vi "Z to circle.vi"(8 "Error In":errorcluster, 10 "Plot points":i32=90, 11 "Z":cdb[](array[numeric])) -> (0 "Error Out":errorcluster, 1 "y0":dbl, 2 "x0":dbl, 3 "plot":cluster{"Array":dbl[], "Array":dbl[]}, 4 "r":dbl format="%.2f", 5 "theta":dbl)   [LabVIEW 2016]
uses:
  <vilib>/gmath/NI_Gmath.lvlib
panel:
  out "Circle fit":cluster{"Array":dbl[], "Array":dbl[]}[](graph)
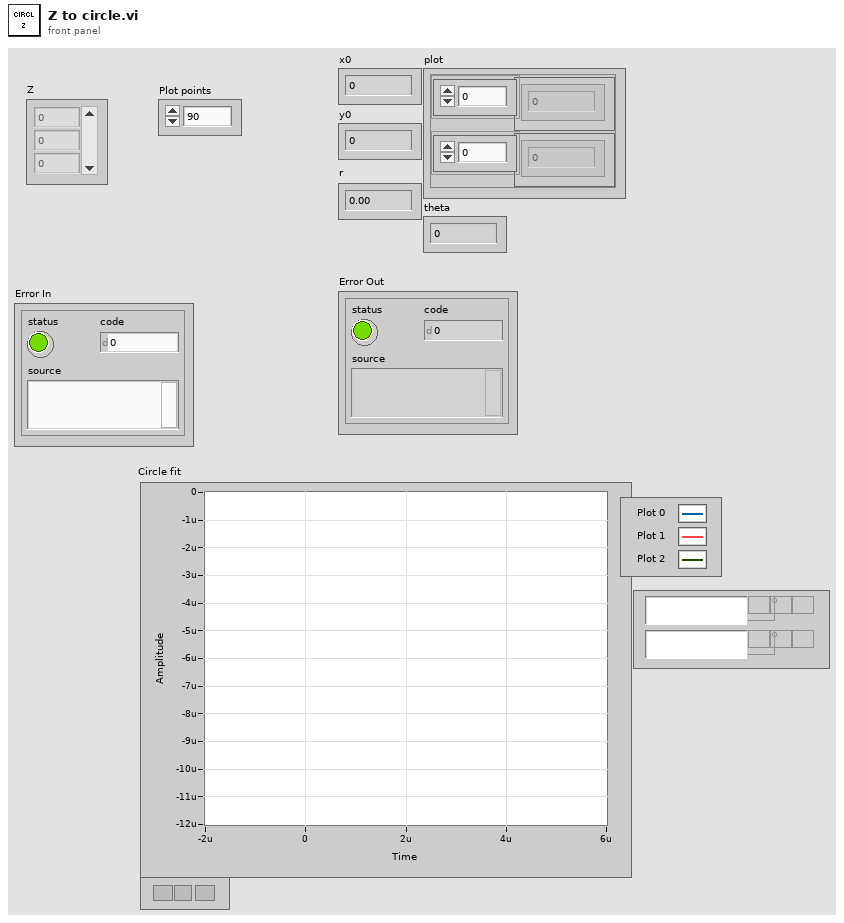
[diagram p1: front panel]
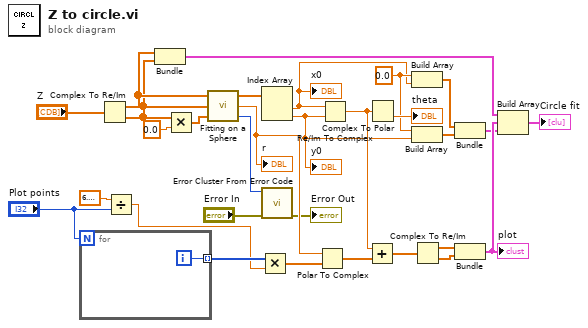
[diagram p0: block diagram]
diagram:
  w4 = 0.0
  n1 = for {
    N: "Plot points" -> [_]
    tunnel: [w31] -> w28 mode=indexing
    i -> [w31]
  }
  n2 = Complex To Re/Im(x + iy="Z") -> (x=w10:dbl[], y=w9:dbl[])
  n3 = Divide(x=6.283185307179586, y="Plot points") -> (x/y=w25:dbl)
  n4 = Bundle(w10, w9) -> (w8:cluster{dbl[], dbl[]})  [unwired: 1 in]
  n5 = Multiply(x=w9, y=0.0) -> (x*y=w30:dbl[])
  n6 = call <vilib>:"Fitting on a Sphere.vi"("Z"=w30, "Y"=w9, "X"=w10) -> ("error"=w16:i32, "r"=w23:dbl, "x0, y0, z0"=w22:dbl[])
  "r" <- w23
  n7 = Multiply(x=w28, y=w25) -> (x*y=w24:dbl[])
  n8 = Index Array(array=w22) -> (element #1=w3:dbl, element #2=w2:dbl)  [unwired: 2 in]
  "x0" <- w3
  "y0" <- w2
  n9 = call <vilib>:"Error Cluster From Error Code.vi"("error in (no error)"="Error In", "error code (0)"=w16) -> ("error out"=→"Error Out":errorcluster)  [unwired: 7 in]
  n10 = Polar To Complex(1:w24, 2:w23) -> (0:w21:cdb[])
  n11 = Re/Im To Complex(1:w2, 2:w3) -> (0:w13:cdb)
  n12 = Add(x=w13, y=w21) -> (x+y=w20:cdb[])
  n13 = Complex To Polar(r * e^(i*theta)=w13) -> (theta=→"theta":dbl)  [unwired: 1 out]
  n14 = Build Array(w4, w3) -> (w5:dbl[])
  n15 = Build Array(w4, w2) -> (w6:dbl[])
  n16 = Complex To Re/Im(x + iy=w20) -> (x=w19:dbl[], y=w18:dbl[])
  n17 = Bundle(w5, w6) -> (w1:cluster{dbl[], dbl[]})  [unwired: 1 in]
  n18 = Bundle(w19, w18) -> (w7:cluster{dbl[], dbl[]})  [unwired: 1 in]
  "plot" <- w7
  n19 = Build Array(w8, w7, w1) -> (→"Circle fit":cluster{dbl[], dbl[]}[])
